vi "Create.vi"(9 "Actor":refnum<class "Actor.lvclass">, 10 "Self Alias":string, 11 "Base Actor in":refnum<class "Base Actor.lvclass">) -> (3 "Base Actor out":refnum<class "Base Actor.lvclass">)   [LabVIEW 2020, in "jettl.lvlib" / "Actor.lvlib" / "Base Actor.lvclass"]
uses:
  Base Actor.lvclass
  Error/Error.lvlib
  Actor/Actor.lvclass
  Msg/Msg.lvclass
  Implemented Msgs.ctl
  Actor.lvlib
  Attributes.ctl
  Created Init.ctl
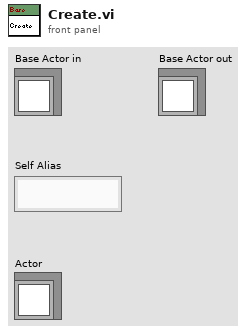
[diagram p1: front panel]
types:
  T1 = typedef "jettl.lvlib/Actor.lvlib/Created Aliases.ctl" = set{string}
  T2 = typedef "jettl.lvlib/Actor.lvlib/Created Init.ctl" = cluster{"Created Attributes":T3, "Is Normal":bool, "Actor":refnum<class "Actor.lvclass">}
  T3 = typedef "jettl.lvlib/Actor.lvlib/Attributes.ctl" = cluster{"Alias":string, "Address":refnum<user-event>, "Implemented Msgs":T4, "Path":path}
  T4 = typedef "jettl.lvlib/Actor.lvlib/Implemented Msgs.ctl" = set{refnum<class "Msg.lvclass">}
  T5 = typedef "jettl.lvlib/Actor.lvlib/Alias to Created Attributes.ctl" = map{string, T3}
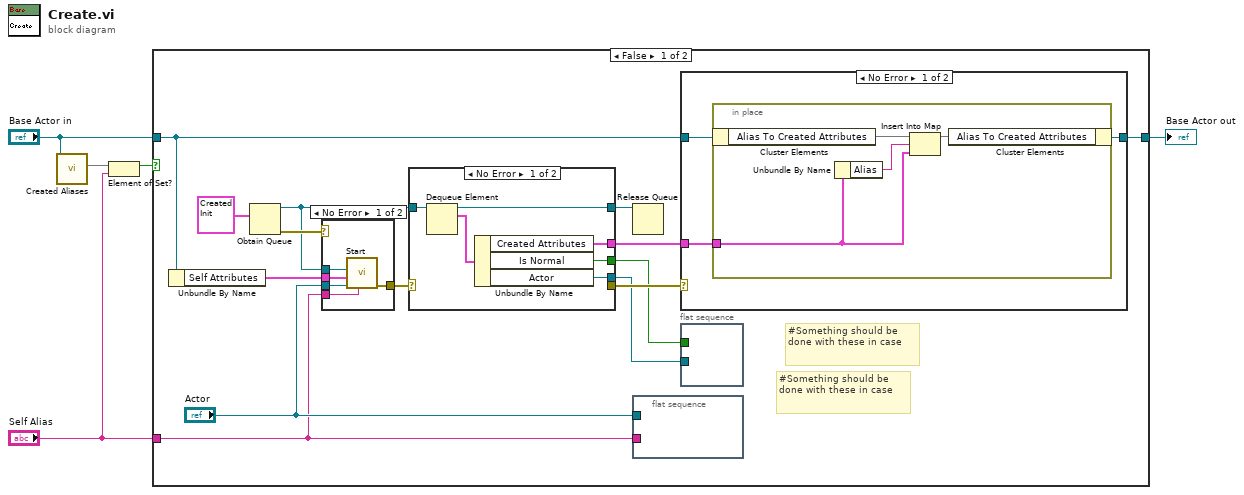
[diagram p0: block diagram]
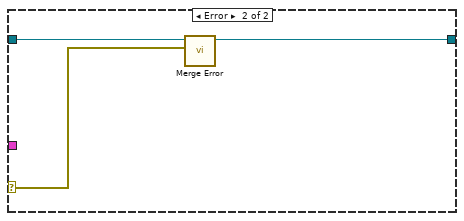
[diagram p4: hidden frame]
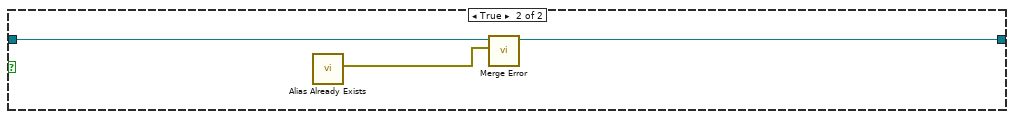
[diagram p5: hidden frame]
diagram:
  n1 = call-dynamic "Created Aliases.vi"("Base Actor in"="Base Actor in") -> ("Created Aliases"=w3:T1)  [unwired: 10 in]
  n2 = Element of Set?(10:"Self Alias", 11:w3) -> (3:w1:bool)
  n3 = case shown="False" w1 {
    tunnel: "Base Actor in" -> [w15 w45]
    tunnel: "Self Alias" -> [w10 _]
    tunnel: [w19 w44] -> w5
    frame False {
      # "#Something should be done with these in case"
      # "#Something should be done with these in case"
      n4 = Unbundle By Name(w15) -> ("Self Attributes"=w13:T3)
      n5 = Obtain Queue(element data type=T2 {"Created Attributes"={"Alias"="", "Address"=refnum, "Implemented Msgs"={}, "Path"=path ""}, "Is Normal"=FALSE, "Actor"=refnum} ("Created Init")) -> (queue out=w12:refnum<queue>, error out=w18:errorcluster)  [unwired: 4 in, 1 out]
      n6 = case shown="No Error" w18 {
        selector: w18 -> [_ w25]
        tunnel: [w24 w25] -> w16
        tunnel: w10 -> [w22 _]
        tunnel: w13 -> [w20 _]
        tunnel: w12 -> [w23 _]
        tunnel: "Actor" -> [w21 _]
        frame No Error {
          n7 = call "Start.vi"("Self Alias"=w22, "Actor"=w21, "Creator Attributes"=w20, "Queue of Created Init"=w23) -> ("error out"=w24:errorcluster)  [unwired: 7 in]
        }
        frame Error {
        }
      }
      n8 = case shown="No Error" w16 {
        selector: w16 -> [_ w33]
        tunnel: [_ w33] -> w17
        tunnel: w12 -> [w31 w32]
        tunnel: [w30 w32] -> w14
        tunnel: [w27 _] -> w7
        tunnel: [w28 _] -> w9
        tunnel: [w26 _] -> w8
        frame No Error {
          n9 = Dequeue Element(queue=w31) -> (queue out=w30:refnum<queue>, element=w29:T2)  [unwired: 2 in, 2 out]
          n10 = Unbundle By Name(w29) -> ("Created Attributes"=w28:T3, "Is Normal"=w27:bool, "Actor"=w26:refnum<class "Actor.lvclass">)
        }
        frame Error {
        }
      }
      n11 = Release Queue(queue=w14) -> ()  [unwired: 2 in, 3 out]
      n12 = flat-sequence {
        tunnel: "Actor" -> [_]
        tunnel: w10 -> [_]
        frame #0 {
        }
      }
      n13 = case shown="No Error" w17 {
        selector: w17 -> [_ w43]
        tunnel: w15 -> [w36 w42]
        tunnel: [w35 w41] -> w19
        tunnel: w9 -> [w34 _]
        frame No Error {
          n14 = in-place {
            in-place-border: w34 -> [w38]
            n15 = in-place-cluster #1(w36) -> ("Alias To Created Attributes"=w40:T5)
            n16 = Unbundle By Name(w38) -> ("Alias"=w37:string)
            n17 = Insert Into Map(map in=w40, key=w37, value=w38) -> (map out=w39:T5)  [unwired: 2 out]
            n18 = in-place-cluster #1("Alias To Created Attributes"=w39) -> (w35:refnum<class "Base Actor.lvclass">)
          }
        }
        frame Error {
          n19 = call-dynamic "Merge Error.vi"("Error"=w43, "Base Actor in"=w42) -> ("Base Actor out"=w41:refnum<class "Base Actor.lvclass">)  [unwired: 9 in]
        }
      }
      n20 = flat-sequence {
        tunnel: w8 -> [_]
        tunnel: w7 -> [_]
        frame #0 {
        }
      }
    }
    frame True {
      n21 = call "Alias Already Exists.vi"() -> ("Error"=w46:errorcluster)  [unwired: 11 in]
      n22 = call-dynamic "Merge Error.vi"("Error"=w46, "Base Actor in"=w45) -> ("Base Actor out"=w44:refnum<class "Base Actor.lvclass">)  [unwired: 9 in]
    }
  }
  "Base Actor out" <- w5
